vi "GUI_ThorlabsWFS.vi"() -> ()   [LabVIEW 2020]
uses:
  Shared/GUI_Template/GUI_master/tcp_new_data_event.ctl
  Shared/GUI_Template/GUI_master/tcp new data cluster.ctl
  <vilib>/vision/Image Controls.llb/IMAQ Image.ctl
panel:
  out "Saturated::1":enum16{"on", "off"}(ring) caption="Saturated"
  out "LowPower::1":enum16{"on", "off"}(ring) caption="LowPower"
  out "SpotfieldImage::1":T1(plugin-control) caption="SpotField"
  out "tcp data event 2":T2
  in  "UDP error message":string
  in  "Refresh Button":bool
  out "GUIdevice 1":string="FrogHPD"
  in  "Tab Control":T3(tab)
  in  "TriggerDelay::1":dbl=0.001 caption="Trigger Delay" min=0.0 max=12.0 format="%_4p"
  in  "Exposure::1":dbl=0.001 caption="Exposure" min=0.0 max=100.0 format="%_4p"
  in  "Select device":string(combo)="U_GhostWFS"
  in  "Trigger::1":enum16{"on", "off"}(ring) caption="trigger"
  in  "PupilToBeam::1":enum16{"on", "off"}(ring) caption="Set Pupil to Beam"
  out "Power too high":bool
  out "Power too low":bool
  in  "PupilXCent::1":dbl=0.001 caption="PupilXCent" min=0.0 max=12.0 format="%_4p"
  in  "PupilYCent::1":dbl=0.001 caption="PupilYCent" min=0.0 max=12.0 format="%_4p"
  in  "PupilXDiam::1":dbl=0.001 caption="PupilXDiam" min=0.0 max=12.0 format="%_4p"
  in  "PupilYDiam::1":dbl=0.001 caption="PupilYDiam" min=0.0 max=12.0 format="%_4p"
  out "RadiusOfCurvature::1":dbl=0.001 caption="Radius of Curvature" min=0.0 max=0.0 format="%_4p"
  out "Zernike3::1":dbl=0.001 caption="Zernike3" min=0.0 max=0.0 format="%_4p"
  out "Image::1":T1(plugin-control) caption="Wavefront"
  in  "stop":bool
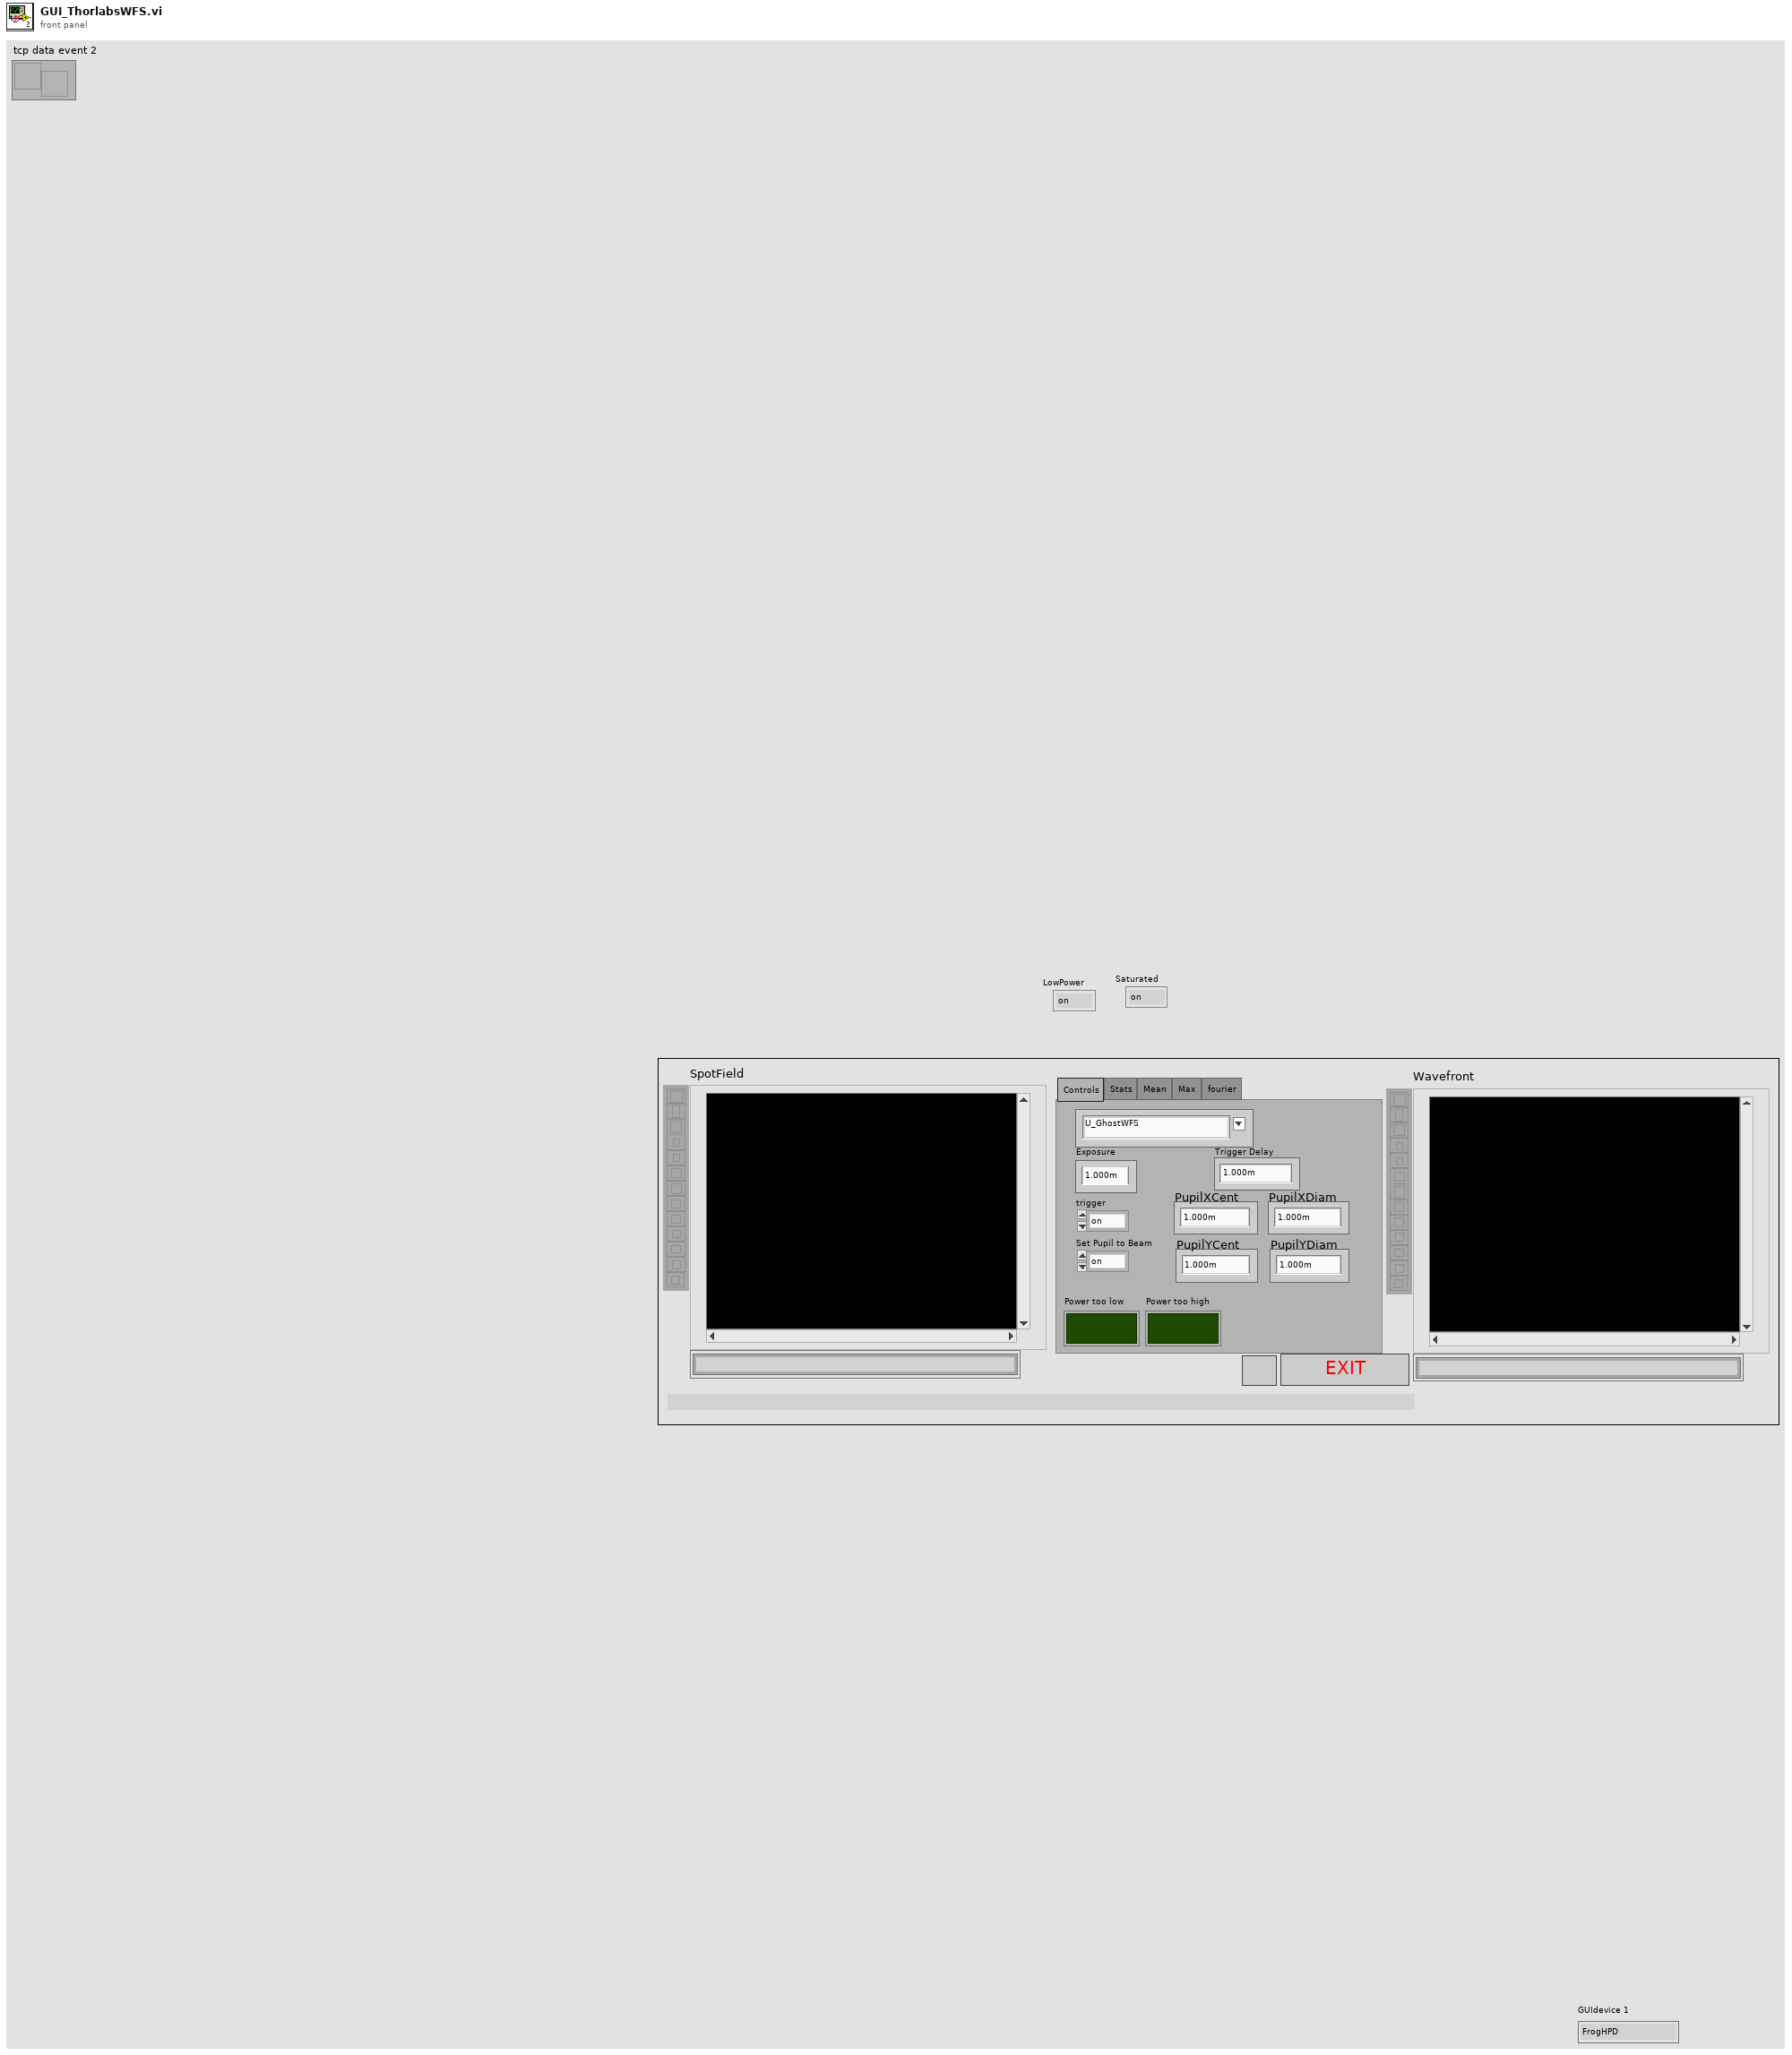
[diagram p1: front panel]
types:
  T1 = typedef "IMAQ Image.ctl" = refnum<image>
  T2 = typedef "tcp_new_data_event.ctl" = refnum<user-event>
  T3 = enum32{"Controls", "Stats", "Mean", "Max", "fourier"}
  T4 = enum32{"invalid app kind", "Development System", "Run Time System", "Student Edition", "Embedded LabVIEW", "Evaluation", "Custom"}
  T5 = typedef "tcp new data cluster.ctl" = cluster{"EventEnum":enum16{"new data", "connection status update"}, "Device name":string}
  T6 = enum32{"Invalid", "Standard", "Closed", "Hidden", "Minimized", "Maximized"}
  T7 = cluster{"Core":cluster{"Current VI Reference":refnum<vi>, "Close Panel on Exit?":bool}, "Your Boolean data":bool, "Your string data":string, "SuperGUI":cluster{"STOP queue":refnum<queue>, "SuperGUI ref":refnum<vi>, "event reg":refnum<event-registration>}, "Images":cluster{"Image::1":T1, "SpotfieldImage::1":T1}}
  T8 = cluster{"STOP queue":refnum<queue>, "SuperGUI ref":refnum<vi>, "event reg":refnum<event-registration>}
  T9 = cluster{"Current VI Reference":refnum<vi>, "Close Panel on Exit?":bool}
  T10 = typedef "Image Type" = u32
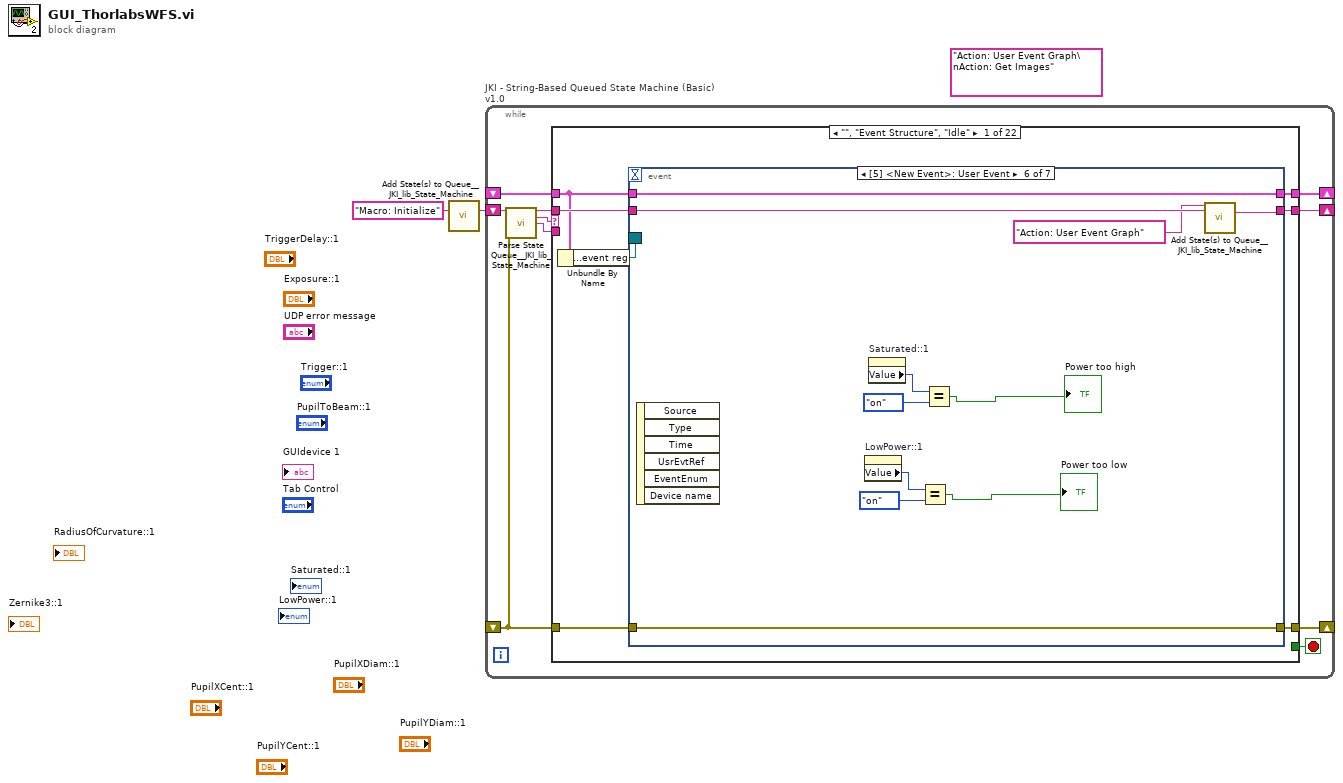
[diagram p0: block diagram]
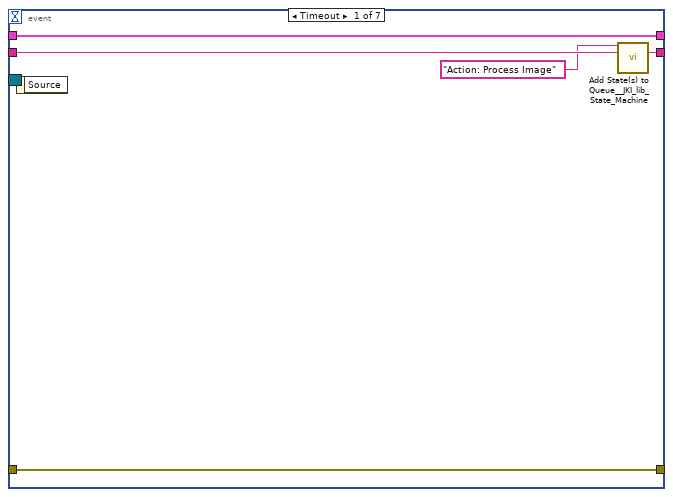
[diagram p2: hidden frame]
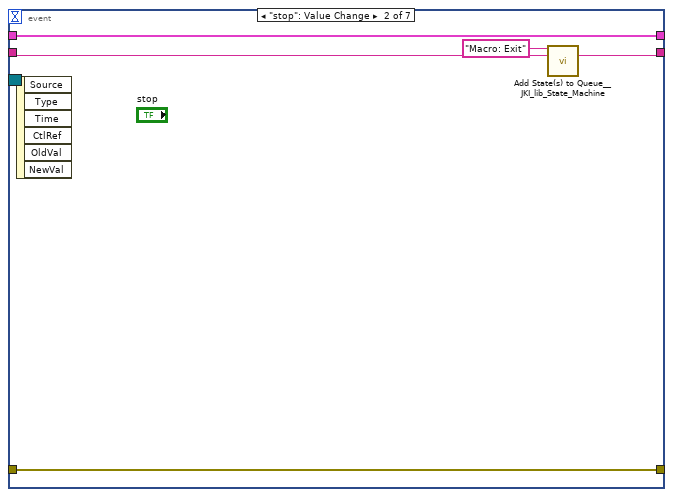
[diagram p3: hidden frame]
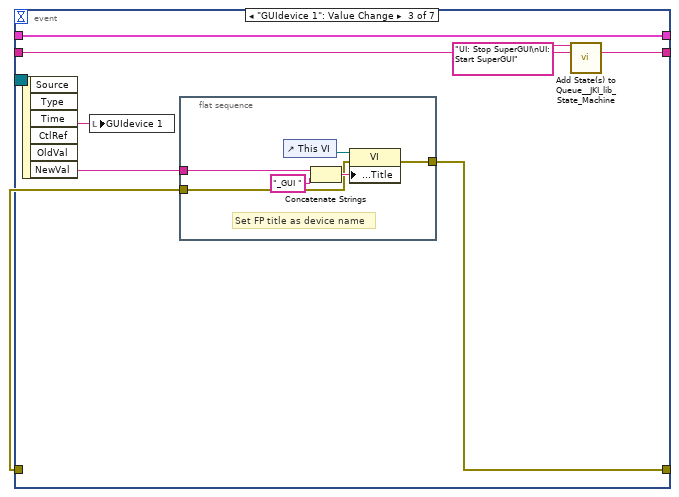
[diagram p4: hidden frame]
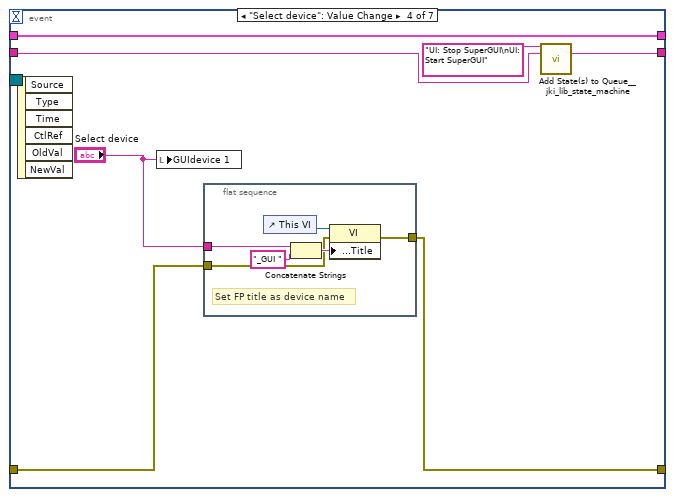
[diagram p5: hidden frame]
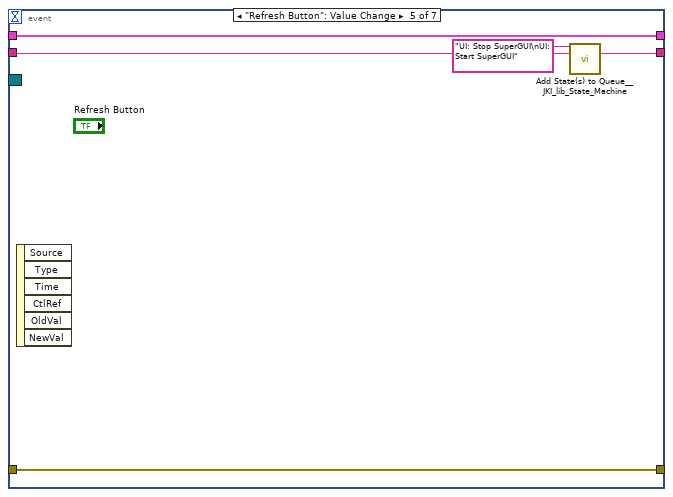
[diagram p6: hidden frame]
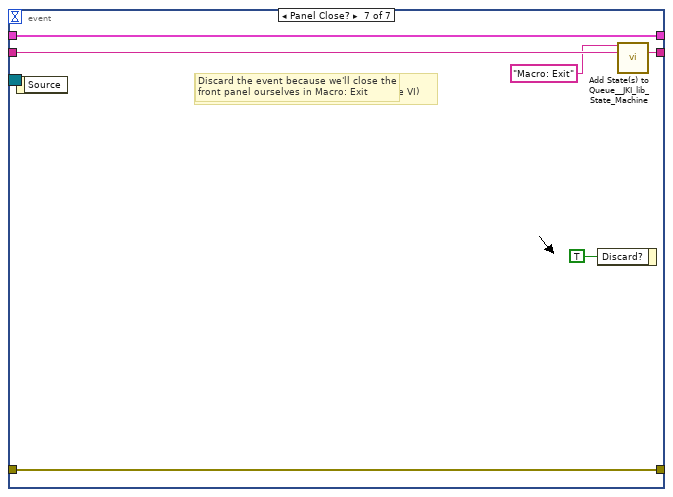
[diagram p7: hidden frame]
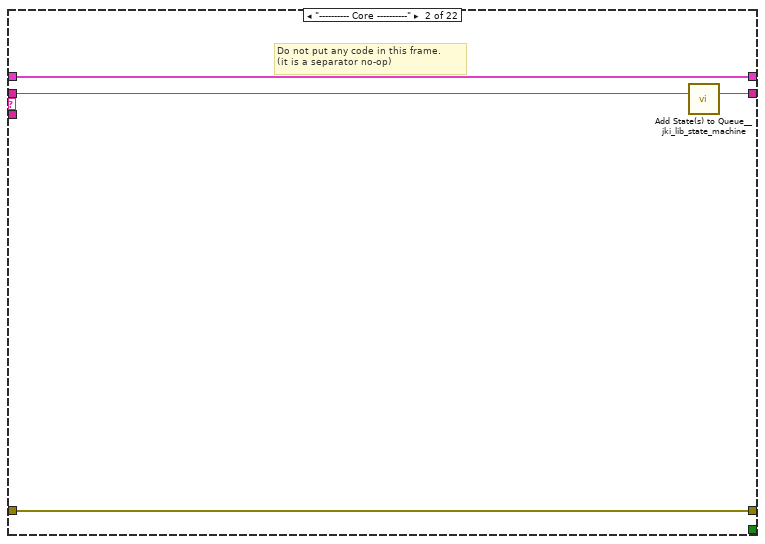
[diagram p8: hidden frame]
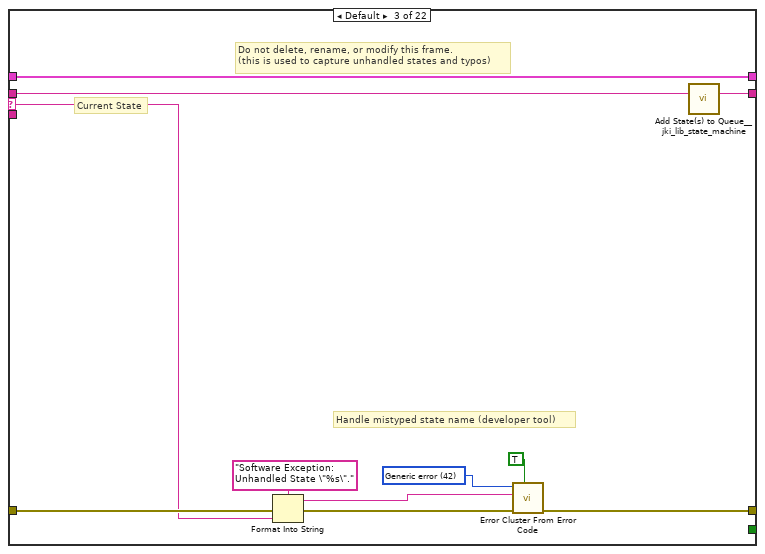
[diagram p9: hidden frame]
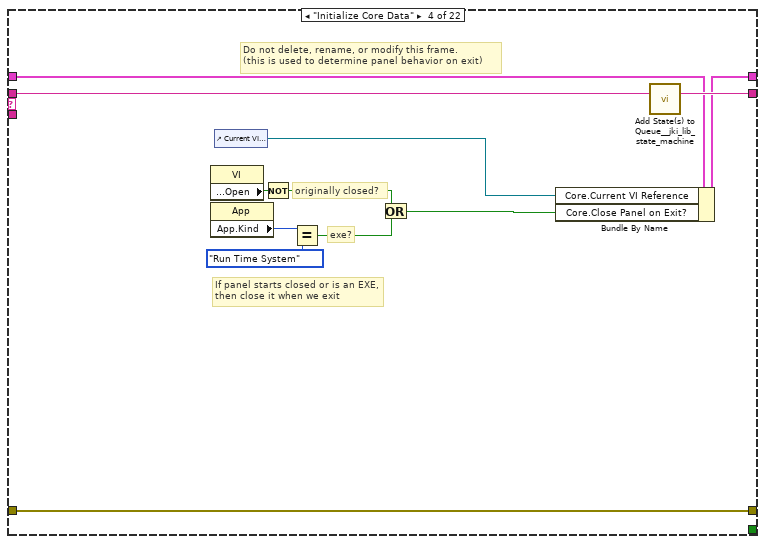
[diagram p10: hidden frame]
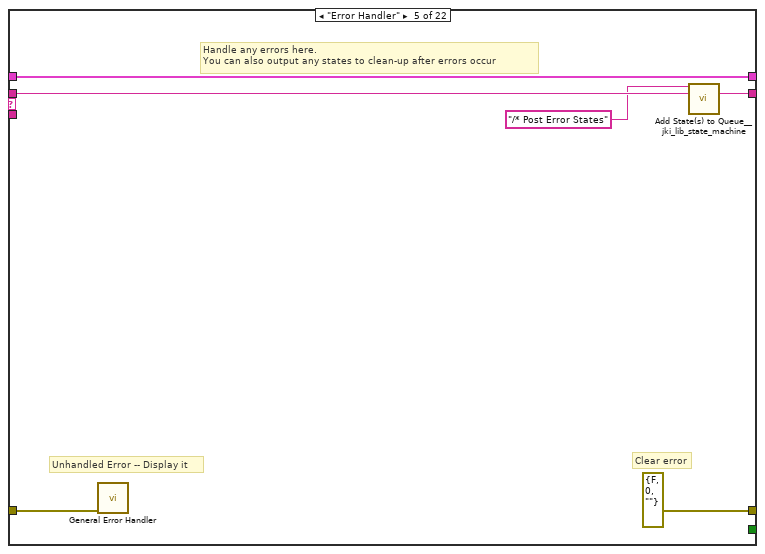
[diagram p11: hidden frame]
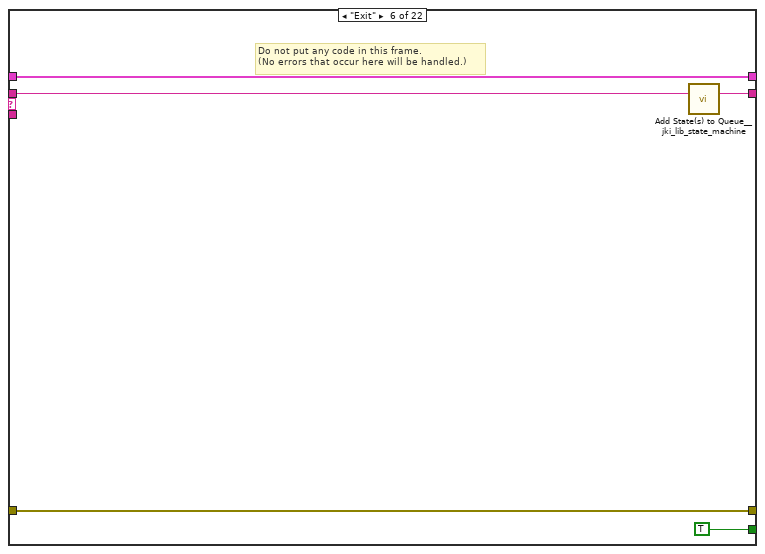
[diagram p12: hidden frame]
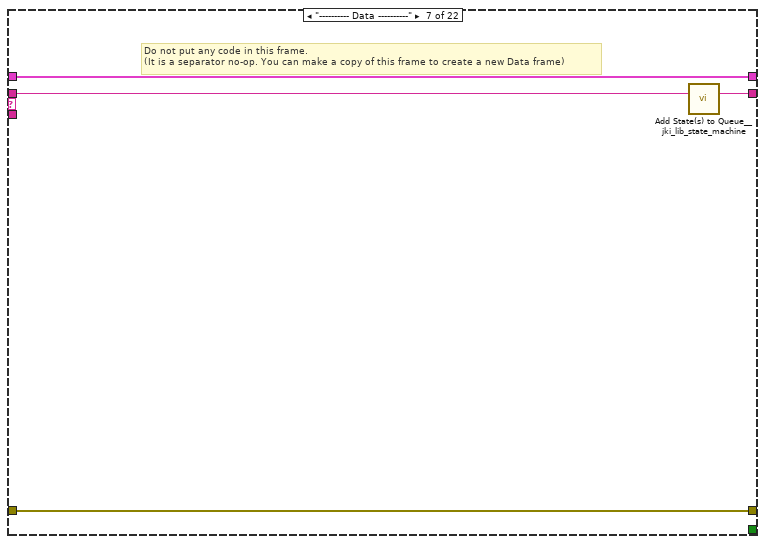
[diagram p13: hidden frame]
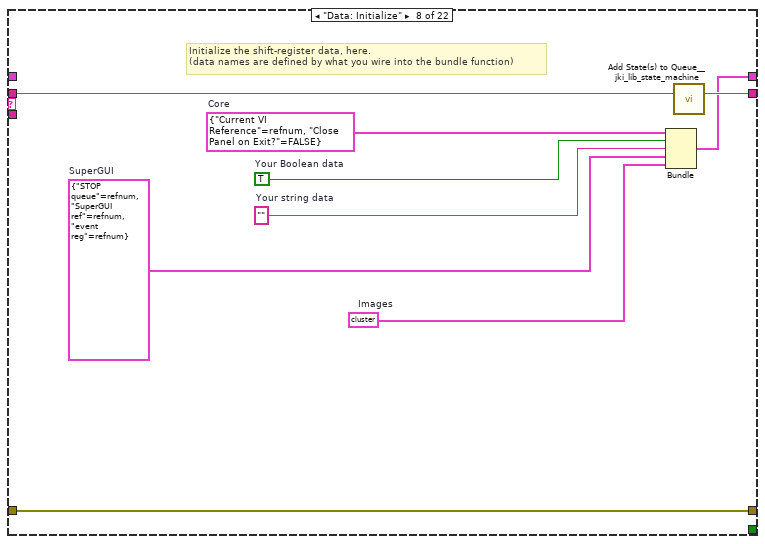
[diagram p14: hidden frame]
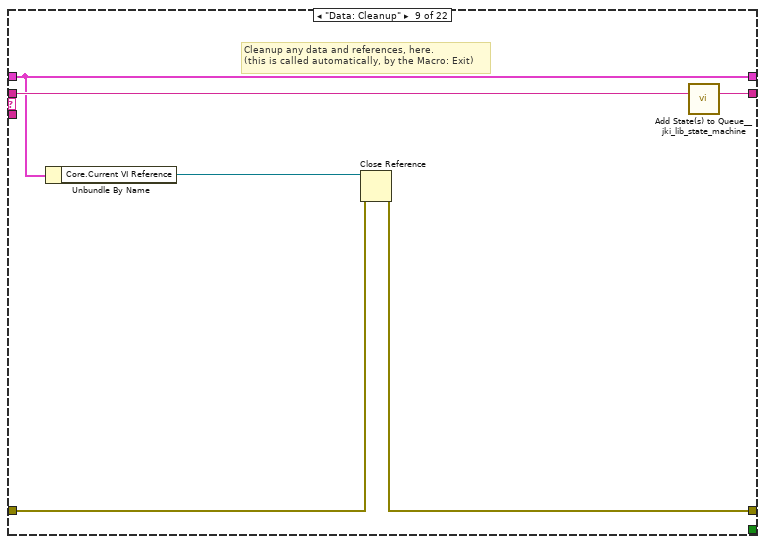
[diagram p15: hidden frame]
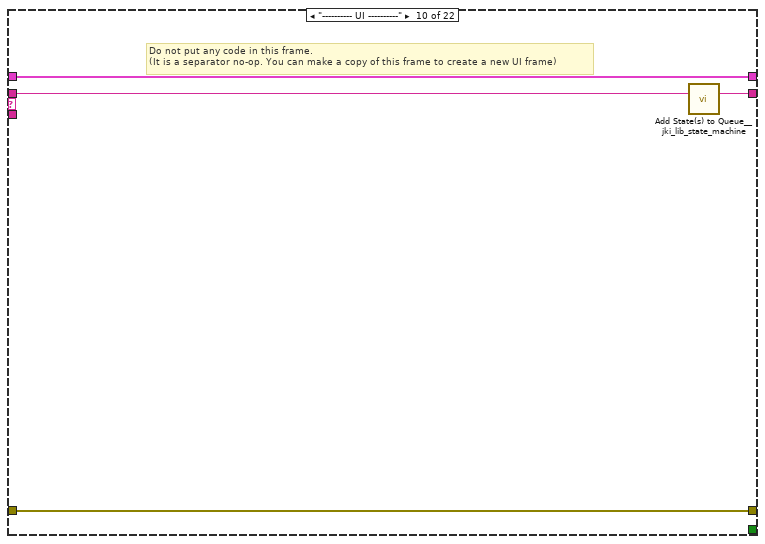
[diagram p16: hidden frame]
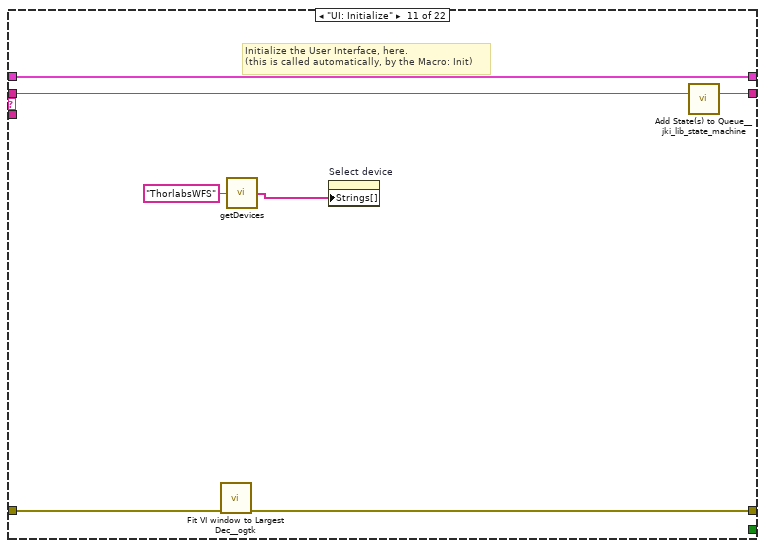
[diagram p17: hidden frame]
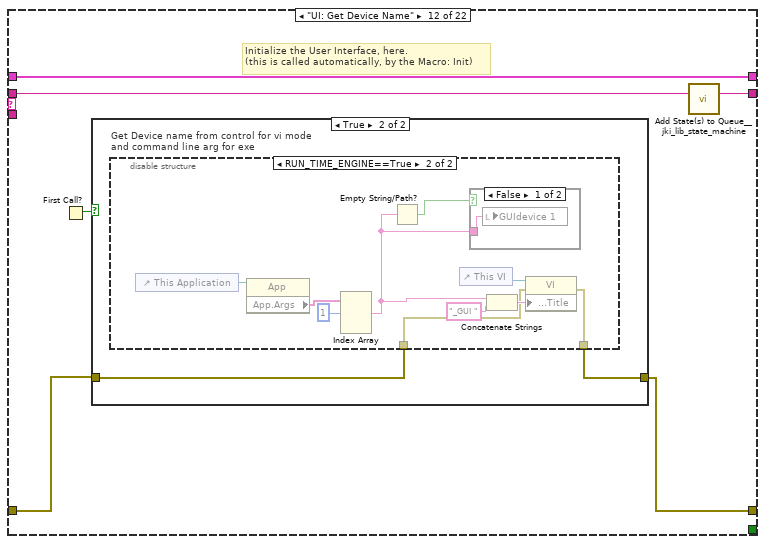
[diagram p18: hidden frame]
diagram:
  (unwired) "Action: User Event Graph\nAction: Get Images" ("State(s) in Front (\"\")")
  n1 = call <vilib>:"Add State(s) to Queue__JKI_lib_State_Machine.vi"("State(s) in (\"\")"="Macro: Initialize") -> ("States Out"=w2:string)  [unwired: 14 in]
  n2 = while "JKI - String-Based Queued State Machine (Basic) v1.0" {
    shift-right: [w5] -> _
    shift-left: _ -> [w4]
    shift-right: [w8] -> _
    shift-left: _ -> [w3]
    shift-right: [w7] -> _
    shift-left: w2 -> [w9]
    stop <- w6 stop-if-true
    n3 = call <vilib>:"Parse State Queue__JKI_lib_State_Machine.vi"("State Queue"=w9, "Error In (no error)"=w3) -> ("Remaining States"=w11:string, "Current State"=w12:string, "Arguments"=w10:string)  [unwired: 11 in]
    n4 = case shown="\"\", \"Event Structure\", \"Idle\"" w12 {
      selector: w12 -> [_ _ w82 _ _ _ _ _ _ _ _ _ _ _ _ _ _ _ _ _ _ _]
      tunnel: w11 -> [w19 w81 w86 w104 w110 w115 w119 w128 w134 w138 w145 w151 w188 w196 w202 w213 w239 w244 w254 w258 w262 w273]
      tunnel: w10 -> [_ _ _ _ _ _ _ _ _ _ _ _ _ _ w197 w207 _ _ _ _ _ _]
      tunnel: w4 -> [w14 w78 w84 w95 w107 w113 w116 _ w129 w135 w143 w149 w179 w191 w200 w209 w236 w241 w251 w255 w259 w268]
      tunnel: [w17 w79 w88 w101 errorcluster {"status"=FALSE, "code"=0, "source"=""} ("error out") w112 w117 w125 w130 w136 w141 w146 w173 w189 w198 w210 w237 w242 w252 w256 w260 w271] -> w8
      tunnel: w3 -> [w16 w79 w87 w101 w106 w112 w117 w125 w131 w136 w142 w147 w174 w190 w199 w211 w237 w242 w252 w256 w260 w271]
      tunnel: [w18 w80 w85 w103 w109 w114 w118 w127 w133 w137 w144 w150 w187 w195 w201 w212 w238 w243 w253 w257 w261 w272] -> w7
      tunnel: [_ _ _ _ _ TRUE _ _ _ _ _ _ _ _ _ _ _ _ _ _ _ _] -> w6
      tunnel: [w15 w78 w84 w102 w107 w113 w116 w126 w129 w135 w143 w149 w178 w191 w200 w209 w236 w241 w251 w255 w259 w267] -> w5
      frame "", "Event Structure", "Idle" {
        n5 = Unbundle By Name(w14) -> ("SuperGUI.event reg"=w13:refnum<event-registration>)
        n6 = event shown="[5] <New Event>: User Event" {
          selector: w13 -> [_ _ _ _ _ _ _]
          dyn-events: _ -> [_ _ _ _ _ _ _]
          timeout: _ -> [_ _ _ _ _ _ _]
          tunnel: w19 -> [w24 w27 w33 w45 w58 w70 w77]
          tunnel: [w23 w26 w32 w44 w57 w69 w76] -> w18
          tunnel: w14 -> [w21 w29 w36 w49 w60 w71 w74]
          tunnel: [w22 w28 w34 w47 w59 w67 w75] -> w17
          tunnel: w16 -> [w22 w28 w35 w48 w59 w67 w75]
          tunnel: [w21 w29 w36 w49 w60 w71 w74] -> w15
          event Timeout {
            n7 = event-data() -> ()  [unwired: 1 in, 1 out]
            n8 = call <vilib>:"Add State(s) to Queue__JKI_lib_State_Machine.vi"("State(s) in Front (\"\")"="Action: Process Image" ("State(s) in Front (\"\")"), "State(s) in (\"\")"=w24) -> ("States Out"=w23:string)  [unwired: 13 in]
          }
          event "stop": Value Change {
            n9 = event-data() -> ()  [unwired: 1 in, 6 out]
            n10 = call <vilib>:"Add State(s) to Queue__JKI_lib_State_Machine.vi"("State(s) in Front (\"\")"="Macro: Exit", "State(s) in (\"\")"=w27) -> ("States Out"=w26:string)  [unwired: 13 in]
          }
          event "GUIdevice 1": Value Change {
            n11 = event-data() -> ("NewVal"=w30:string)  [unwired: 1 in, 5 out]
            n12 = local write "GUIdevice 1"(w30) -> ()
            n13 = flat-sequence {
              tunnel: [w39] -> w34
              tunnel: w35 -> [w38]
              tunnel: w30 -> [w37]
              frame #0 {
                # "Set FP title as device name"
                n14 = control-ref of="This VI"() -> (w42:refnum<vi>)
                n15 = Concatenate Strings(w37, "_GUI ") -> (w41:string)
                n16 = property class="VI"(reference=w42, error in=w38, "Front Panel.Title"=w41) -> (error out=w39:errorcluster)  [unwired: 1 out]
              }
            }
            n17 = call <vilib>:"Add State(s) to Queue__JKI_lib_State_Machine.vi"("State(s) in Front (\"\")"="UI: Stop SuperGUI\nUI: Start SuperGUI", "State(s) in (\"\")"=w33) -> ("States Out"=w32:string)  [unwired: 13 in]
          }
          event "Select device": Value Change {
            n18 = event-data() -> ()  [unwired: 1 in, 6 out]
            n19 = local write "GUIdevice 1"("Select device") -> ()
            n20 = flat-sequence {
              tunnel: [w52] -> w47
              tunnel: w48 -> [w51]
              tunnel: "Select device" -> [w50]
              frame #0 {
                # "Set FP title as device name"
                n21 = control-ref of="This VI"() -> (w55:refnum<vi>)
                n22 = Concatenate Strings(w50, "_GUI ") -> (w54:string)
                n23 = property class="VI"(reference=w55, error in=w51, "Front Panel.Title"=w54) -> (error out=w52:errorcluster)  [unwired: 1 out]
              }
            }
            n24 = call <vilib>:"Add State(s) to Queue__jki_lib_state_machine.vi"("State(s) in Front (\"\")"="UI: Stop SuperGUI\nUI: Start SuperGUI", "State(s) in (\"\")"=w45) -> ("States Out"=w44:string)  [unwired: 13 in]
          }
          event "Refresh Button": Value Change {
            n25 = event-data() -> ()  [unwired: 1 in, 6 out]
            n26 = call <vilib>:"Add State(s) to Queue__JKI_lib_State_Machine.vi"("State(s) in Front (\"\")"="UI: Stop SuperGUI\nUI: Start SuperGUI", "State(s) in (\"\")"=w58) -> ("States Out"=w57:string)  [unwired: 13 in]
          }
          event User Event {
            n27 = event-data() -> ()  [unwired: 1 in, 6 out]
            n28 = property on="LowPower::1" class="Enum (strict)"() -> ("Value"=w62:enum16{"on", "off"})  [unwired: 2 in, 2 out]
            n29 = property on="Saturated::1" class="Enum (strict)"() -> ("Value"=w65:enum16{"on", "off"})  [unwired: 2 in, 2 out]
            n30 = Equal?(x=w62, y=enum16{"on"}."on") -> (x = y?=→"Power too low":bool)
            n31 = Equal?(x=w65, y=enum16{"on"}."on") -> (x = y?=→"Power too high":bool)
            n32 = call <vilib>:"Add State(s) to Queue__JKI_lib_State_Machine.vi"("State(s) in Front (\"\")"="Action: User Event Graph" ("State(s) in Front (\"\")"), "State(s) in (\"\")"=w70) -> ("States Out"=w69:string)  [unwired: 13 in]
          }
          event Panel Close? {
            # "Discard the event because we'll close the front panel ourselves in Macro: Exit"
            # "Close Panel button (pressed) Event\n(this executes Macro: Exit to terminate the VI)"
            n33 = event-data() -> ()  [unwired: 1 in, 1 out]
            n34 = event-data("Discard?"=TRUE) -> ()  [unwired: 1 in, 1 out]
            n35 = call <vilib>:"Add State(s) to Queue__JKI_lib_State_Machine.vi"("State(s) in Front (\"\")"="Macro: Exit", "State(s) in (\"\")"=w77) -> ("States Out"=w76:string)  [unwired: 13 in]
          }
        }
      }
      frame "---------- Core ----------" {
        # "Do not put any code in this frame.\n(it is a separator no-op)"
        n36 = call <vilib>:"Add State(s) to Queue__jki_lib_state_machine.vi"("State(s) in (\"\")"=w81) -> ("States Out"=w80:string)  [unwired: 14 in]
      }
      frame Default {
        w91 = 42 items=["No error", "Argument error", "Memory is full", "Out of zone", "End of file", "File already open", "Generic file I/O error", "File not found", "File permission error", "Disk is full", "Duplicate path", "Too many files open", "System feature not enabled", "Resource file not found", "Cannot add resource", "Resource not found", "Image not found", "Image memory error", "Pen does not exist", "Config type invalid", "Config token not found", "Config parse error", "Config memory error", "Bad external code format", "Bad external code offset", "External code not present", "Null window", "Destroy window error", "Null menu", "Print aborted", "Bad print record", "Print driver error", "Windows error during printing", "Memory error during printing", "Print dialog error", "Generic print error", "Invalid device refnum", "Device not found", "Device parameter error", "Device unit error", "Cannot open device", "Device call aborted", "Generic error", "Cancelled by user", "Object ID too low", "Object ID too high", "Object not in heap", "Unknown heap", "Unknown object (invalid DefProc)", "Unknown object (DefProc not in table)", "Message out of range", "Invalid (null) method", "Unknown message", "Manager call not supported", "Bad address", "Network operation in progress", "Network operation timed out", "Connection is busy", "Network attribute not supported", "Network error", "Address in use", "System out of memory", "Connection aborted", "Connection refused", "Not connected", "Already connected", "Connection closed", "Initialization error (interapplication manager)", "Bad occurrence", "Wait on unbound occurrence handler", "Occurrence queue overflow", "Datalog type conflict", "Unused", "Unrecognized type (interapplication manager)", "Memory corrupt", "Failed to make temporary DLL", "Old CIN version", "Drag socket not found", "Failed to load drop-object", "Failed to register OLE object", "Failed to release OLE object", "Format specifier type mismatch", "Unknown format specifier", "Too few format specifiers", "Too many format specifiers", "Scan failed", "Newer CIN version", "Error converting to variant", "Runtime menu error", "Password tampered", "Variant attribute not found", "Incompatible variant data type", "Event data is not available", "Event Store is not present", "Occurrence is not found", "Event Queue is not created", "Event info is not available", "Refnum passed is NULL", "Error retrieving Class GUID", "Error retrieving CoClass GUID", "Error retrieving TypeLib GUID.", "Bad built application magic bytes.", "Specific driver is different from the specific driver associated with the Logical Name.", "There is no session opened to the class driver.", "Max Error", "MAX - Error with config objects", "MAX - Error loading configuration", "MAX - Group not supported"]
        # "Current State"
        # "Do not delete, rename, or modify this frame.\n(this is used to capture unhandled states and typos)"
        # "Handle mistyped state name (developer tool)"
        n37 = Format Into String(format string="Software Exception: Unhandled State \"%s\"." ("message"), error in=w87, w82) -> (resulting string=w90:string, error out=w89:errorcluster)  [unwired: 1 in]
        n38 = call <vilib>:"Error Cluster From Error Code.vi"("show call chain? (False)"=TRUE, "error in (no error)"=w89, "error message (\"\")"=w90, "error code (0)"=w91) -> ("error out"=w88:errorcluster)  [unwired: 5 in]
        n39 = call <vilib>:"Add State(s) to Queue__jki_lib_state_machine.vi"("State(s) in (\"\")"=w86) -> ("States Out"=w85:string)  [unwired: 14 in]
      }
      frame "Initialize Core Data" {
        # "Do not delete, rename, or modify this frame.\n(this is used to determine panel behavior on exit)"
        # "originally closed?"
        # "exe?"
        # "If panel starts closed or is an EXE, then close it when we exit"
        n40 = property class="VI"() -> ("Front Panel.Open"=w100:bool)  [unwired: 2 in, 2 out]
        n41 = property class="App"() -> ("App.Kind"=w99:T4)  [unwired: 2 in, 2 out]
        n42 = control-ref of="Current VI Reference"() -> (w93:refnum<vi>)
        n43 = Not(x=w100) -> (.not. x?=w97:bool)
        n44 = Equal?(x=w99, y=T4."Run Time System" ("Application:Kind")) -> (x = y?=w96:bool)
        n45 = Or(x=w97, y=w96) -> (x .or. y?=w94:bool)
        n46 = Bundle By Name(cluster=w95, "Core.Current VI Reference"=w93, "Core.Close Panel on Exit?"=w94) -> (w102:T7)
        n47 = call <vilib>:"Add State(s) to Queue__jki_lib_state_machine.vi"("State(s) in (\"\")"=w104) -> ("States Out"=w103:string)  [unwired: 14 in]
      }
      frame "Error Handler" {
        # "Unhandled Error -- Display it"
        # "Handle any errors here.\nYou can also output any states to clean-up after errors occur"
        # "Clear error"
        n48 = call <vilib>:"General Error Handler.vi"("error in (no error)"=w106) -> ()  [unwired: 10 in, 5 out]
        n49 = call <vilib>:"Add State(s) to Queue__jki_lib_state_machine.vi"("State(s) in Front (\"\")"="/* Post Error States", "State(s) in (\"\")"=w110) -> ("States Out"=w109:string)  [unwired: 13 in]
      }
      frame "Exit" {
        # "Do not put any code in this frame.\n(No errors that occur here will be handled.)"
        n50 = call <vilib>:"Add State(s) to Queue__jki_lib_state_machine.vi"("State(s) in (\"\")"=w115) -> ("States Out"=w114:string)  [unwired: 14 in]
      }
      frame "---------- Data ----------" {
        # "Do not put any code in this frame.\n(It is a separator no-op. You can make a copy of this frame to create a new Data frame)"
        n51 = call <vilib>:"Add State(s) to Queue__jki_lib_state_machine.vi"("State(s) in (\"\")"=w119) -> ("States Out"=w118:string)  [unwired: 14 in]
      }
      frame "Data: Initialize" {
        w120 = cluster{"Image::1":T1, "SpotfieldImage::1":T1} {"Image::1"="remote image 0000000014FE4274", "SpotfieldImage::1"="remote image 0000000014FE4274"}  # Images
        w121 = T8 {"STOP queue"=refnum, "SuperGUI ref"=refnum, "event reg"=refnum}  # SuperGUI
        w122 = T9 {"Current VI Reference"=refnum, "Close Panel on Exit?"=FALSE}  # Core
        w124 = TRUE  # Your Boolean data
        w123 = ""  # Your string data
        # "Initialize the shift-register data, here.\n(data names are defined by what you wire into the bundle function)"
        n52 = Bundle("Core"=w122, "Your Boolean data"=w124, "Your string data"=w123, "SuperGUI"=w121, "Images"=w120) -> (w126:T7)  [unwired: 1 in]
        n53 = call <vilib>:"Add State(s) to Queue__jki_lib_state_machine.vi"("State(s) in (\"\")"=w128) -> ("States Out"=w127:string)  [unwired: 14 in]
      }
      frame "Data: Cleanup" {
        # "Cleanup any data and references, here.\n(this is called automatically, by the Macro: Exit)"
        n54 = Unbundle By Name(w129) -> ("Core.Current VI Reference"=w132:refnum<vi>)
        n55 = Close Reference(reference=w132, error in (no error)=w131) -> (error out=w130:errorcluster)
        n56 = call <vilib>:"Add State(s) to Queue__jki_lib_state_machine.vi"("State(s) in (\"\")"=w134) -> ("States Out"=w133:string)  [unwired: 14 in]
      }
      frame "---------- UI ----------" {
        # "Do not put any code in this frame.\n(It is a separator no-op. You can make a copy of this frame to create a new UI frame)"
        n57 = call <vilib>:"Add State(s) to Queue__jki_lib_state_machine.vi"("State(s) in (\"\")"=w138) -> ("States Out"=w137:string)  [unwired: 14 in]
      }
      frame "UI: Initialize" {
        # "Initialize the User Interface, here.\n(this is called automatically, by the Macro: Init)"
        n58 = call <userlib>:"Fit VI window to Largest Dec__ogtk.vi"("error in (no error)"=w142) -> ("error out"=w141:errorcluster)  [unwired: 5 in, 1 out]
        n59 = call "getDevices.vi"("Device Class"="ThorlabsWFS") -> ("All Devices"=w139:string[])
        n60 = property on="Select device" class="CmbBox"("Strings[]"=w139) -> ()  [unwired: 2 in, 2 out]
        n61 = call <vilib>:"Add State(s) to Queue__jki_lib_state_machine.vi"("State(s) in (\"\")"=w145) -> ("States Out"=w144:string)  [unwired: 14 in]
      }
      frame "UI: Get Device Name" {
        # "Initialize the User Interface, here.\n(this is called automatically, by the Macro: Init)"
        n62 = First Call?() -> (First Call?: T/F=w148:bool)
        n63 = case shown="True" w148 {
          tunnel: w147 -> [w152 w154]
          tunnel: [w152 w153] -> w146
          frame False {
          }
          frame True {
            n64 = disable-structure "Get Device name from control for vi mode\nand command line arg for exe" shown="RUN_TIME_ENGINE==True" {
              disable-tunnel: w154 -> [w155 w157]
              disable-tunnel: [w155 w156] -> w153
              frame condition #0 (active) {
              }
              frame condition #1 {
                n65 = control-ref of="This Application"() -> (w165:refnum<vi>)
                n66 = property class="App"(reference=w165) -> ("App.Args"=w164:string[])  [unwired: 1 in, 2 out]
                n67 = Index Array(array=w164, index #1=1 ("index")) -> (element #1=w158:string)  [unwired: 2 in, 2 out]
                n68 = Empty String/Path?(string/path=w158) -> (empty?=w162:bool)
                n69 = control-ref of="This VI"() -> (w161:refnum<vi>)
                n70 = case shown="False" w162 {
                  tunnel: w158 -> [w166 _]
                  frame False {
                    n71 = local write "GUIdevice 1"(w166) -> ()
                  }
                  frame True {
                  }
                }
                n72 = Concatenate Strings(w158, "_GUI ") -> (w160:string)
                n73 = property class="VI"(reference=w161, error in=w157, "Front Panel.Title"=w160) -> (error out=w156:errorcluster)  [unwired: 1 out]
              }
            }
          }
        }
        n74 = call <vilib>:"Add State(s) to Queue__jki_lib_state_machine.vi"("State(s) in (\"\")"=w151) -> ("States Out"=w150:string)  [unwired: 14 in]
      }
      frame "UI: Start SuperGUI" {
        # "create stop queue for supergui and its clones"
        # "x100 abort will be dependent on caller VI\nx80 abort will be independent of caller vi, this will abort vi when labview is closed."
        # "Start SuperGUI asynchronous way"
        n75 = vi-ref "GUI_Master_subvi_reentrant_queues.vi"() -> (w172:refnum<vi>)
        n76 = property class="VI"(reference=w172) -> ("Path"=w171:path)  [unwired: 1 in, 2 out]
        n77 = Create User Event(user event datatype=T5 {"EventEnum"=enum."new data", "Device name"="Device name"} ("New Event"), error in=w174) -> (user event=w169:refnum<user-event>, error out=w180:errorcluster)
        "tcp data event 2" <- w169
        n78 = control-ref of="This Application"() -> (w177:refnum<vi>)
        n79 = control-ref of="This VI"() -> (w176:refnum<vi>)
        n80 = Open VI Reference(type specifier VI Refnum (for type only)=refnum<vi> refnum, vi path=w171, options=256) -> (vi reference=w186:refnum<vi>, error out=w185:errorcluster)  [unwired: 3 in]
        n81 = register-events(w169) -> (reference out=w168:refnum<event-registration>)  [unwired: 2 in, 1 out]
        n82 = call "supergui create stop queue.vi"() -> ("STOP Queue out"=w182:refnum<queue>)  [unwired: 11 in]
        n83 = Current VI's Menubar() -> (w175:refnum<k9>)
        n84 = call-by-ref "Start Asynchronous Call"(reference=w186, error in=w185, "STOP Queue in"=w182, "This Application"=w177, 8:"error in (no error)"=w180, "tcp data event"=w169, "Caller menu reference"=w175, "Caller VI ref"=w176) -> (reference out=w170:refnum<vi>, error out=w173:errorcluster)  [unwired: 5 in, 1 out]
        n85 = Bundle By Name(cluster=w179, "SuperGUI.event reg"=w168, "SuperGUI.SuperGUI ref"=w170, "SuperGUI.STOP queue"=w182) -> (w178:T7)
        n86 = call <vilib>:"Add State(s) to Queue__jki_lib_state_machine.vi"("State(s) in Front (\"\")"="Action: Get Images" ("State(s) in Front (\"\")"), "State(s) in (\"\")"=w188) -> ("States Out"=w187:string)  [unwired: 13 in]
      }
      frame "UI: Stop SuperGUI" {
        # "Stop Supergui Clone and wait until it exit properly"
        n87 = Unbundle By Name(w191) -> ("SuperGUI.SuperGUI ref"=w193:refnum<vi>, "SuperGUI.STOP queue"=w192:refnum<queue>)
        n88 = Release Queue(queue=w192, error in (no error)=w190) -> (error out=w194:errorcluster)  [unwired: 1 in, 2 out]
        n89 = call-by-ref "Wait On Asynchronous Call"(reference=w193, error in=w194) -> ("error out"=w189:errorcluster)  [unwired: 11 in, 2 out]
        n90 = call <vilib>:"Add State(s) to Queue__jki_lib_state_machine.vi"("State(s) in (\"\")"=w196) -> ("States Out"=w195:string)  [unwired: 14 in]
      }
      frame "UI: Cursor Set" {
        # "Argument"
        # "Set and Unset Cursor Busy.\n(Usage: \"UI: Cursor Set >> Busy|Idle\")"
        n91 = case shown="\"Idle\", Default" w197 {
          tunnel: w199 -> [w204 w206]
          tunnel: [w203 w205] -> w198
          frame "Idle", Default {
            n92 = call <vilib>:"Unset Busy.vi"("error in (no error)"=w204) -> ("error out"=w203:errorcluster)  [unwired: 10 in]
          }
          frame "Busy" {
            n93 = call <vilib>:"Set Busy.vi"("error in (no error)"=w206) -> ("error out"=w205:errorcluster)  [unwired: 9 in, 1 out]
          }
        }
        n94 = call <vilib>:"Add State(s) to Queue__jki_lib_state_machine.vi"("State(s) in (\"\")"=w202) -> ("States Out"=w201:string)  [unwired: 14 in]
      }
      frame "UI: Front Panel State" {
        # "Argument"
        # "Set Front Panel Open or Closed\n(Usage: \"UI: Front Panel State >> Open|Close\")"
        n95 = Unbundle By Name(w209) -> ("Core.Current VI Reference"=w208:refnum<vi>)
        n96 = case shown="\"Open\", Default" w207 {
          tunnel: w211 -> [w217 w230]
          tunnel: [w219 w231] -> w210
          tunnel: w208 -> [w218 w228]
          frame "Open", Default {
            n97 = property class="VI"(reference=w218, error in=w217) -> (reference out=w215:refnum<vi>, error out=w216:errorcluster, "Front Panel.Open"=w214:bool)
            n98 = case shown="False" w214 {
              tunnel: [w222 w225] -> w219
              tunnel: w216 -> [w221 w225]
              tunnel: w215 -> [w220 _]
              frame False {
                n99 = invoke class="VI" method="FP.Open"(reference=w220, error in=w221, "Activate"=TRUE, "State"=T6."Standard") -> (error out=w222:errorcluster)  [unwired: 1 in, 4 out]
              }
              frame True {
              }
            }
          }
          frame "Close" {
            n100 = property class="VI"(reference=w228, error in=w230) -> (reference out=w227:refnum<vi>, error out=w229:errorcluster, "Front Panel.Open"=w226:bool)
            n101 = case shown="True" w226 {
              tunnel: [w232 w235] -> w231
              tunnel: w229 -> [w232 w234]
              tunnel: w227 -> [_ w233]
              frame False {
              }
              frame True {
                n102 = invoke class="VI" method="FP.Close"(reference=w233, error in=w234) -> (error out=w235:errorcluster)  [unwired: 1 in, 2 out]
              }
            }
          }
        }
        n103 = call <vilib>:"Add State(s) to Queue__jki_lib_state_machine.vi"("State(s) in (\"\")"=w213) -> ("States Out"=w212:string)  [unwired: 14 in]
      }
      frame "---------- Macro ----------" {
        # "Do not put any code in this frame.\n(It is a separator no-op. You can make a copy of this frame to create a new Macro frame)"
        n104 = call <vilib>:"Add State(s) to Queue__jki_lib_state_machine.vi"("State(s) in (\"\")"=w239) -> ("States Out"=w238:string)  [unwired: 14 in]
      }
      frame "Macro: Initialize" {
        # "Initialization Macro\n(This is called once, when the VI starts)"
        n105 = call <vilib>:"Add State(s) to Queue__jki_lib_state_machine.vi"("State(s) in Front (\"\")"="Data: Initialize\nInitialize Core Data\nUI: Initialize\nUI: Get Device Name\nUI: Start SuperGUI\nUI: Front Panel State >> Open", "State(s) in (\"\")"=w244) -> ("States Out"=w243:string)  [unwired: 13 in]
      }
      frame "Macro: Exit" {
        # "Exit Macro\n(This is called once, when the VI exits)"
        n106 = Unbundle By Name(w251) -> ("Core.Close Panel on Exit?"=w250:bool)
        n107 = Select(t="UI: Front Panel State >> Close", s=w250, f="") -> (s? t:f=w247:string)
        n108 = call <vilib>:"Add State(s) to Queue__jki_lib_state_machine.vi"("State(s) in (\"\")"=w247, "State(s) at Back (\"\")"="Data: Cleanup\nExit") -> ("States Out"=w245:string)  [unwired: 13 in]
        n109 = call <vilib>:"Add State(s) to Queue__jki_lib_state_machine.vi"("State(s) in Front (\"\")"=w245, "State(s) in (\"\")"=w254) -> ("States Out"=w253:string)  [unwired: 13 in]
      }
      frame "---------- New Category ----------" {
        # "Template Separator\n(You can make a copy of, or modify, this frame)"
        n110 = call <vilib>:"Add State(s) to Queue__jki_lib_state_machine.vi"("State(s) in (\"\")"=w258) -> ("States Out"=w257:string)  [unwired: 14 in]
      }
      frame "Action: User Event Graph" {
        n111 = call <vilib>:"Add State(s) to Queue__jki_lib_state_machine.vi"("State(s) in (\"\")"=w262) -> ("States Out"=w261:string)  [unwired: 14 in]
      }
      frame "Action: Get Images" {
        w264 = T10 0 items=["Grayscale (U8)", "Grayscale (I16)", "Grayscale (SGL)", "Complex (CSG)", "RGB (U32)", "HSL (U32)", "RGB (U64)", "Grayscale (U16)"] ("Image Type")
        w269 = T10 7 items=["Grayscale (U8)", "Grayscale (I16)", "Grayscale (SGL)", "Complex (CSG)", "RGB (U32)", "HSL (U32)", "RGB (U64)", "Grayscale (U16)"] ("Image Type")
        n112 = call "IMAQ Create"("Image Name"="SpotfieldImage::1", "Image Type"=w264) -> ("New Image"=w263:T1)  [unwired: 3 in, 1 out]
        "SpotfieldImage::1" <- w263
        n113 = call "IMAQ Create"("Image Name"="Image::1", "Image Type"=w269) -> ("New Image"=w266:T1)  [unwired: 3 in, 1 out]
        "Image::1" <- w266
        n114 = Bundle By Name(cluster=w268, "Images.Image::1"=w266, "Images.SpotfieldImage::1"=w263) -> (w267:T7)
        n115 = call <vilib>:"Add State(s) to Queue__jki_lib_state_machine.vi"("State(s) in (\"\")"=w273) -> ("States Out"=w272:string)  [unwired: 14 in]
      }
    }
  }
